vi "Import Custom Device Configuration.vi"(8 "error in":errorcluster, 10 "Path":path, 11 "Item Ref in":u64 format="%.0x") -> (0 "error out":errorcluster, 2 "cancelled":bool, 3 "Item Ref out":u64 format="%.0x")   [LabVIEW 2026, in "NIDMM Configuration.lvlib"]
uses:
  NIDMM Configuration.lvlib
  NationalInstruments.VeriStand.SystemDefinitionAPI
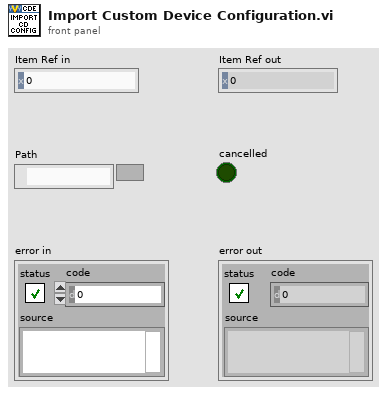
[diagram p1: front panel]
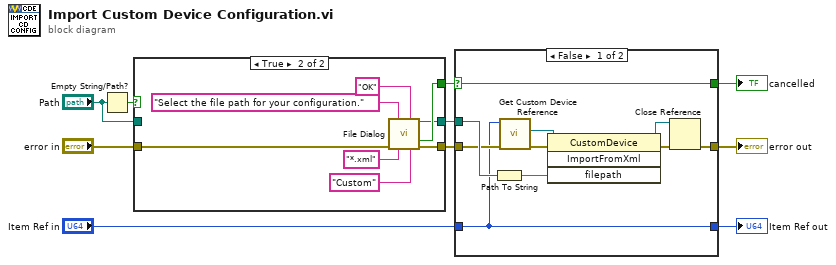
[diagram p0: block diagram]
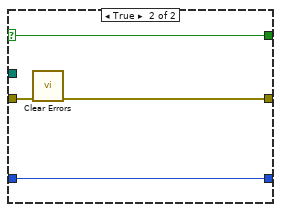
[diagram p2: hidden frame]
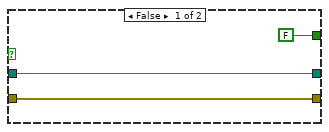
[diagram p3: hidden frame]
diagram:
  n1 = Empty String/Path?(string/path="Path") -> (empty?=w7:bool)
  n2 = case shown="True" w7 {
    tunnel: [FALSE ("cancelled") w16] -> w4
    tunnel: [w13 w21] -> w9
    tunnel: [w11 w15] -> w5
    tunnel: "error in" -> [w13 w20]
    tunnel: "Path" -> [w11 _]
    frame False {
    }
    frame True {
      n3 = call "File Dialog"("prompt"="Select the file path for your configuration.", "button label"="OK", "error in"=w20, "pattern (all files)"="*.xml", "pattern label"="Custom") -> ("selected path"=w15:path, "cancelled"=w16:bool, "error out"=w21:errorcluster)  [unwired: 7 in, 1 out]
    }
  }
  n4 = case shown="False" w4 {
    selector: w4 -> [w27 w33]
    tunnel: [w22 w34] -> w8
    tunnel: w9 -> [w26 w35]
    tunnel: w5 -> [w31 _]
    tunnel: [w27 w33] -> w3
    tunnel: "Item Ref in" -> [w25 w32]
    tunnel: [w25 w32] -> w1
    frame False {
      n5 = Path To String(path=w31) -> (string=w30:string)
      n6 = call "Get Custom Device Reference.vi"("error in"=w26, "Item Ref in"=w25) -> ("error out"=w24:errorcluster, "Custom Device"=w23:refnum<k24>)  [unwired: 7 in, 1 out]
      n7 = invoke class="CustomDevice" method="ImportFromXml"(reference=w23, error in=w24, "filepath"=w30) -> (reference out=w29:refnum<k24>, error out=w28:errorcluster)  [unwired: 1 in, 2 out]
      n8 = Close Reference(reference=w29, error in (no error)=w28) -> (error out=w22:errorcluster)
    }
    frame True {
      n9 = call <vilib>:"Clear Errors.vi"("error in (no error)"=w35) -> ("error out"=w34:errorcluster)  [unwired: 5 in, 1 out]
    }
  }
  "error out" <- w8
  "Item Ref out" <- w1
  "cancelled" <- w3
